vi "PI_TWS.vi"(0 "System no.":i32=1, 2 "Wavepoint":i32[](array[numeric]), 3 "Trigger value":i32[](array[numeric]), 5 "error in":errorcluster) -> (14 "Hidden error":bool, 19 "error out":errorcluster)   [LabVIEW 8.6]
doc: "Sets trigger values for point(s) on the waveform and checks for error. Trigger value is bit-mapped. Hidden error is TRUE if selected system reports error code not equal to 0. \n\nValid for E-710\n\nE-710: Wavepoint can be 1-16000. Trigger value is bitmapped:\n· Bit 0: trigger line 1: 0 not active, 1 active\n· Bit 1: trigger line 2: 0 not active, 1 active\n· Bit 2: trigger line 3: 0 not active, 1 active\n· Bit 3: trigger line 4: 0 not active, 1 active\n· Bit 8: If = 0, then the Trigger values apply to corresponding Wavepoints only.\nIf = 1, then the Trigger value applies to all points between the last point set by this command and the corresponding Wavepoint point."
panel:
  # "Sets trigger values for point(s) on the waveform and checks for\nerror.  \"Trigger value\" is bit-mapped."
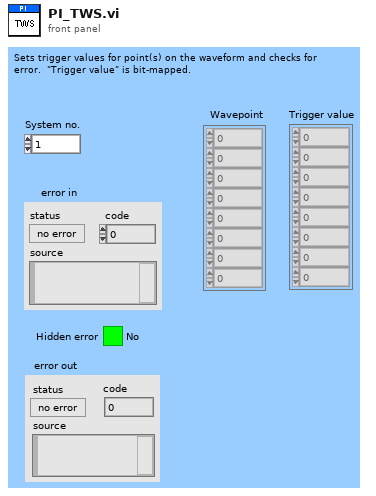
[diagram p1: front panel]
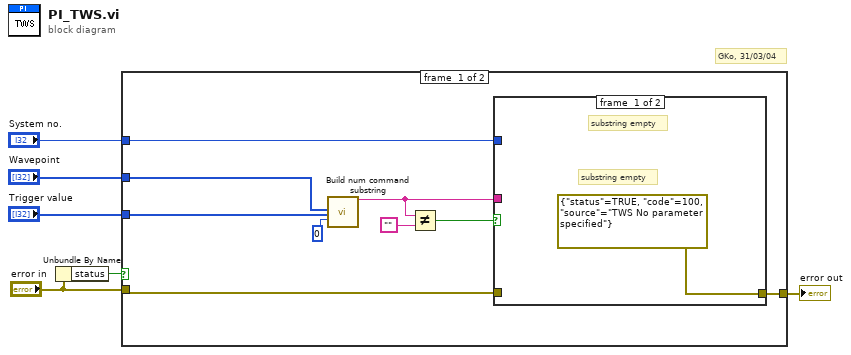
[diagram p0: block diagram]
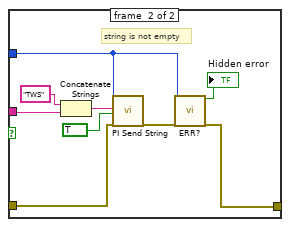
[diagram p2: hidden frame]
diagram:
  # "GKo, 31/03/04"
  n1 = Unbundle By Name("error in") -> ("status"=w2:bool)
  n2 = case shown="False" w2 {
    tunnel: [w15 w26] -> w6
    tunnel: "Trigger value" -> [w12 _]
    tunnel: "error in" -> [w7 w26]
    tunnel: "System no." -> [w11 _]
    tunnel: "Wavepoint" -> [w10 _]
    frame #0 {
      n3 = call "Build num command substring.vi"("Num 1"=w10, "Num 2"=w12, "No. of digits"=i16 0) -> ("Command substring"=w13:string)  [unwired: 16 out]
      n4 = Not Equal?(x=w13, y="") -> (x != y?=w8:bool)
      n5 = case shown="True" w8 {
        tunnel: w13 -> [_ w24]
        tunnel: [errorcluster {"status"=TRUE, "code"=100, "source"="TWS No parameter specified"} ("error out") w19] -> w15
        tunnel: w7 -> [_ w21]
        tunnel: w11 -> [_ w18]
        frame #0 {
          # "substring empty"
          # "substring empty"
        }
        frame #1 {
          # "string is not empty"
          n6 = Concatenate Strings("TWS", w24) -> (w22:string)
          n7 = call "PI Send String.vi"("System no."=w18, "String to send"=w22, "Attach Linefeed?"=TRUE, "error in"=w21) -> ("error out"=w20:errorcluster)  [unwired: 15 out]
          n8 = call "ERR?.vi"("System no."=w18, "error in"=w20) -> ("Hidden error"=→"Hidden error":bool, "error out"=w19:errorcluster)  [unwired: 16 out]
        }
      }
    }
    frame #1 {
    }
  }
  "error out" <- w6
